vi "Auto Arm Pot Controller.vi"(1 "error in":errorcluster, 2 "armSetPoint":dbl format="%.2f") -> (0 "error out":errorcluster)   [LabVIEW 2017]
uses:
  <vilib>/Rock Robotics/WPI/ThirdParty/Phoenix-LabVIEW/Motor Controller/Controls/CTRE_Phoenix_MotorControl_ControlMode.ctl
  <vilib>/Rock Robotics/Network Tables/NT Write Number.vi
  Global Arm Variables.vi
  <vilib>/addons/control/pid/pid.llb/PID (DBL).vi
  <vilib>/addons/control/pid/NI_PID_pid.lvlib
panel:
  out "armPotValue":dbl
  out "armMotorCmd":dbl
  out "potValue-potSetPoint":dbl
  out "'errorSignalMultipledKc":dbl
  out "errorSignal":dbl
  out "Waveform Chart":T1(graph)
  out "dt out (s)":dbl format="%.3f"
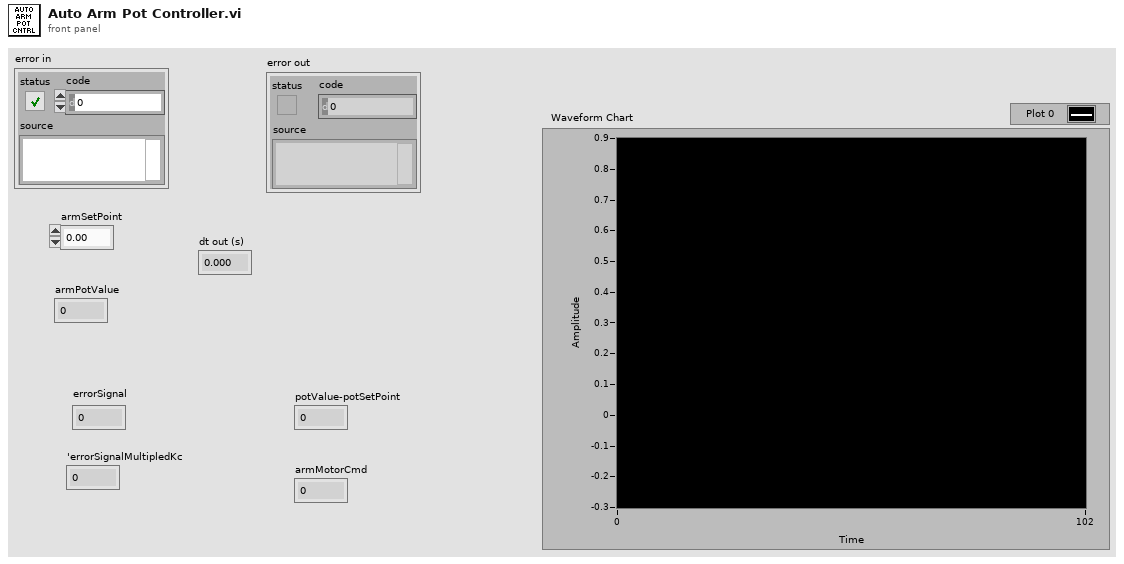
[diagram p1: front panel]
types:
  T1 = cluster{"Normalized Value":dbl, "armSetpoint":dbl, "output":dbl, dbl}
  T2 = cluster{"proportional gain (Kc)":dbl, "integral time (Ti, min)":dbl, "derivative time (Td, min)":dbl}
  T3 = typedef "CTRE_Phoenix_MotorControl_ControlMode.ctl" = u16
  T4 = typedef "WPI_MotorControlDeviceRef.ctl" = cluster{"DeviceStatus":errorcluster, "Type":T5, "PWM":cluster{"PWM Channel":T6, "DeadBand":T7}, "CAN":cluster{"Device Number":u8, "SetOutput VI Ref":variant, "GetOutput VI Ref":variant, "Enable VI Ref":variant, "Disable VI Ref":variant, "Data":variant}, "Invert":bool, "DIO PWM":cluster{"PWM \"Enable\" Channel":T6, "DIOChannel":T8, "PWM Rate":dbl}}
  T5 = typedef "WPI_MotorControlType.ctl" = enum16{"PWM", "CAN", "DIO PWM"}
  T6 = typedef "FPGA_DIOPWMChannel.ctl" = enum8{"PWM 0", "PWM 1", "PWM 2", "PWM 3", "PWM 4", "PWM 5", "PWM 6", "PWM 7", "PWM 8", "PWM 9", "PWM MXP 0", "PWM MXP 1", "PWM MXP 2", "PWM MXP 3", "PWM MXP 4", "PWM MXP 5", "PWM MXP 6", "PWM MXP 7", "PWM MXP 8", "PWM MXP 9", "Invalid"}
  T7 = typedef "WPI_PWMDeadband.ctl" = cluster{"Name":string, "maxPositivePwm":i32, "minPositivePwm":i32, "centerPwm":i32, "maxNegativePwm":i32, "minNegativePwm":i32, "angularRange":u16}
  T8 = typedef "FPGA_DIOChannel.ctl" = enum8{"DIO 0", "DIO 1", "DIO 2", "DIO 3", "DIO 4", "DIO 5", "DIO 6", "DIO 7", "DIO 8", "DIO 9", "DIO MXP 0", "DIO MXP 1", "DIO MXP 2", "DIO MXP 3", "DIO MXP 4", "DIO MXP 5", "DIO MXP 6", "DIO MXP 7", "DIO MXP 8", "DIO MXP 9", "DIO MXP 10", "DIO MXP 11", "DIO MXP 12", "DIO MXP 13", "DIO MXP 14", "DIO MXP 15", "SPI Port CS1", "SPI Port CS2", "SPI Port CS3", "SPI Port MISO", "SPI Port MOSI", "Invalid"}
  T9 = cluster{"armPotValue":dbl, "armSetPoint":dbl, "output":dbl, dbl}
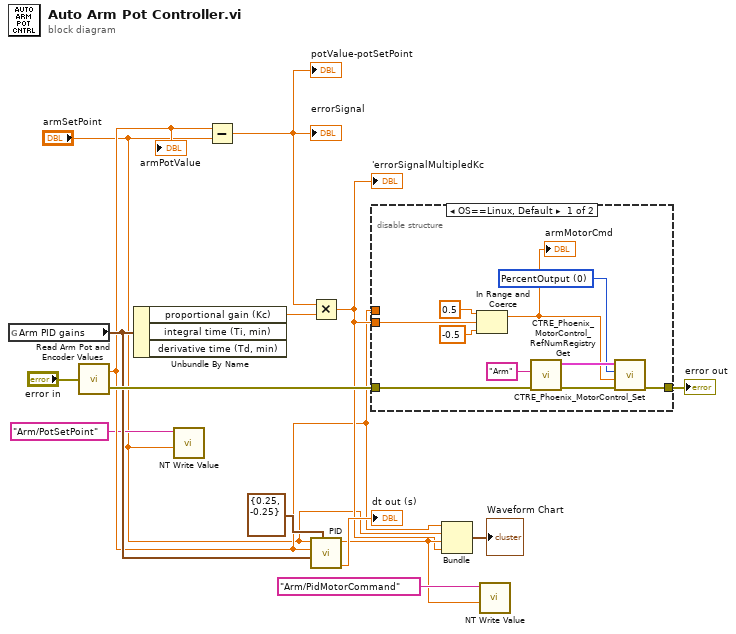
[diagram p0: block diagram]
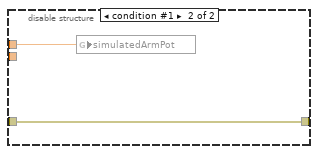
[diagram p2: hidden frame]
diagram:
  n1 = global read "Global Arm Variables.vi" "Arm PID gains"() -> (w4:T2)
  n2 = call "Read Arm Pot and Encoder Values.vi"("error in (no error)"="error in") -> ("armPotValue"=w3:dbl, "error out"=w12:errorcluster)
  "armPotValue" <- w3
  n3 = Unbundle By Name(w4) -> ("proportional gain (Kc)"=w6:dbl)  [unwired: 2 out]
  n4 = call-poly <vilib>:"NT Write Value.vi"("Numeric"="armSetPoint", "Name"="Arm/PotSetPoint") -> ()  [unwired: 9 in, 1 out]
  n5 = Subtract(x=w3, y="armSetPoint") -> (x-y=w7:dbl)
  "errorSignal" <- w7
  "potValue-potSetPoint" <- w7
  n6 = Multiply(x=w7, y=w6) -> (x*y=w5:dbl)
  "'errorSignalMultipledKc" <- w5
  n7 = call-poly <vilib>:"PID.vi"("output range"=cluster{"output high":dbl, "output low":dbl} {"output high"=0.25, "output low"=-0.25}, "PID gains"=w4, "process variable"=w3, "setpoint"="armSetPoint") -> ("dt out (s)"=→"dt out (s)":dbl, "output"=w8:dbl)  [unwired: 6 in]
  n8 = disable-structure shown="OS==Linux, Default" {
    disable-tunnel: [w22 w27] -> w11
    disable-tunnel: w5 -> [w19 _]
    disable-tunnel: w12 -> [w21 w27]
    disable-tunnel: w3 -> [_ w26]
    frame condition #0 (active) {
      w24 = T3 0 items=["PercentOutput"=0, "Position"=1, "Velocity"=2, "Current"=3, "Follower"=5, "MotionProfile"=6, "MotionMagic"=7, "MotionMagicArc"=8, "MotionProfileArc"=10, "Disabled"=15] ("Control Mode")
      n9 = In Range and Coerce(upper limit=0.5, x=w19, lower limit=-0.5) -> (coerced(x)=w16:dbl)  [unwired: 1 out]
      "armMotorCmd" <- w16
      n10 = call <vilib>:"CTRE_Phoenix_MotorControl_RefNumRegistryGet.vi"("error in (no error)"=w21, "refnum name"="Arm" ("Motor ID")) -> ("error out"=w23:errorcluster, "PhoenixMotorControlDevRef"=w25:T4)  [unwired: 8 in]
      n11 = call <vilib>:"CTRE_Phoenix_MotorControl_Set.vi"("error in (no error)"=w23, "Output"=w16, "Control Mode"=w24, "PhoenixMotorControlDevRef"=w25) -> ("error out"=w22:errorcluster)  [unwired: 6 in, 1 out]
    }
    frame condition #1 {
      n12 = global write "Global Arm Variables.vi" "simulatedArmPot"(w26) -> ()
    }
  }
  "error out" <- w11
  n13 = Bundle("armPotValue"=w3, "armSetPoint"="armSetPoint", "output"=w8, w5) -> (→"Waveform Chart":T9)  [unwired: 1 in]
  n14 = call-poly <vilib>:"NT Write Value.vi"("Numeric"=w8, "Name"="Arm/PidMotorCommand") -> ()  [unwired: 9 in, 1 out]
